vi "Agilent Configure Standard Waveform.vi"(6 "Frequency (Hz)":dbl, 7 "Offset (V)":dbl, 8 "error in (no error)":errorcluster, 9 "Amplitude (V)":dbl, 10 "Function":i32(ring) items=["Sine", "Square", "Triangle"], 11 "VISA resource name":refnum<visa-resource-name>) -> (0 "error out":errorcluster, 3 "VISA resource name out":refnum<visa-resource-name>)   [LabVIEW 2014]
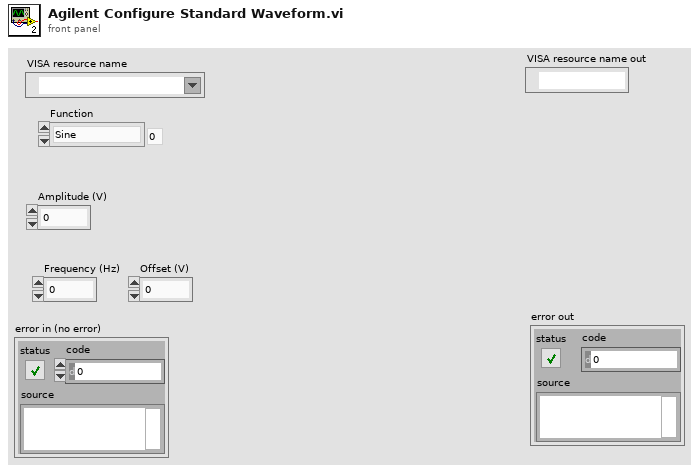
[diagram p1: front panel]
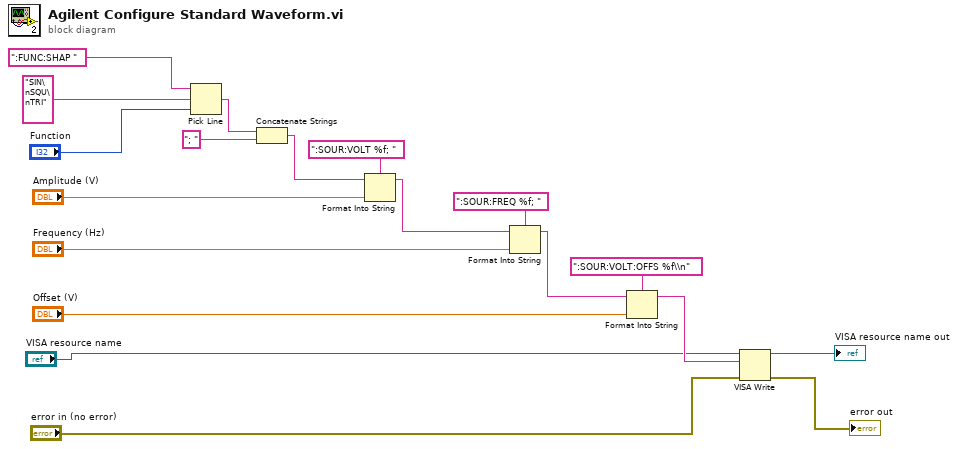
[diagram p0: block diagram]
diagram:
  n1 = Pick Line(string ("")=":FUNC:SHAP ", multi-line string="SIN\nSQU\nTRI", line index="Function") -> (output string=w16:string)
  n2 = Concatenate Strings(w16, "; " ("string")) -> (w13:string)
  n3 = Format Into String(format string=":SOUR:VOLT %f; ", initial string=w13, "Amplitude (V)") -> (resulting string=w7:string)  [unwired: 1 in, 1 out]
  n4 = Format Into String(format string=":SOUR:FREQ %f; ", initial string=w7, "Frequency (Hz)") -> (resulting string=w6:string)  [unwired: 1 in, 1 out]
  n5 = Format Into String(format string=":SOUR:VOLT:OFFS %f\\n", initial string=w6, "Offset (V)") -> (resulting string=w5:string)  [unwired: 1 in, 1 out]
  n6 = VISA Write(VISA resource name="VISA resource name", write buffer=w5, error in (no error)="error in (no error)") -> (VISA resource name out=→"VISA resource name out":refnum<visa-resource-name>, error out=→"error out":errorcluster)  [unwired: 1 out]
